vi "GetIQ_int16.vi"(8 "error in (no error)":errorcluster, 11 "reference in":refnum<class "mmWave data.lvclass">) -> (0 "error out":errorcluster, 1 "dt":dbl, 2 "data":i16[](array[numeric]), 3 "reference out":refnum<class "mmWave data.lvclass">)   [LabVIEW 2019, in "mmWave data.lvclass"]
uses:
  mmWave data.lvclass
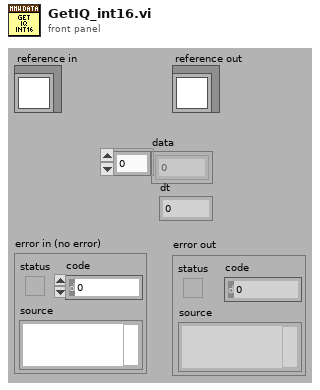
[diagram p1: front panel]
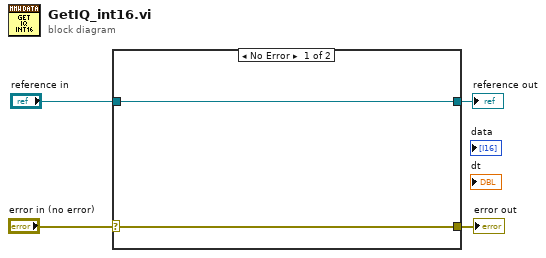
[diagram p0: block diagram]
diagram:
  n1 = case shown="No Error" "error in (no error)" {
    selector: "error in (no error)" -> [w6 w8]
    tunnel: [w6 w8] -> w3
    tunnel: [w5 w7] -> w1
    tunnel: "reference in" -> [w5 w7]
    frame No Error {
    }
    frame Error {
    }
  }
  "error out" <- w3
  "reference out" <- w1
